vi "FS Operation Variable.vi"(9 "Variable":T1, 11 "Feature In":string="FeatureScript 1247;\nimport(path : \"onshape/std/geometry.fs\", version : \"1247.0\");\n\nannotation { \"Feature Type Name\" : \"LabVIEW Feature\" }\nexport const myFeature = defineFeature(function(context is Context, id is Id, definition is map)\n    precondition\n    {\n        // Define the parameters of the feature type\n    }\n    {\n        // Define the function's action\n    });") -> (3 "Feature Out":string="FeatureScript 1247;\nimport(path : \"onshape/std/geometry.fs\", version : \"1247.0\");\n\nannotation { \"Feature Type Name\" : \"LVFeat1\" }\nexport const myFeature = defineFeature(function(context is Context, id is Id, definition is map)\n    precondition\n    {\n        // Define the parameters of the feature type\n    }\n    {\n        // Define the function's action\n\nvar sketch1 = newSketch(context, id + \"sketch1\", {\n                \"sketchPlane\" : qCreatedBy(makeId(\"Top\"), EntityType.FACE)\n        });\n        // Create sketch entities here\n        skRectangle(sketch1, \"rectangle1\", {\n                \"firstCorner\" : vector(0, 0) * inch,\n                \"secondCorner\" : vector(3, 4) * inch\n        });\n        \n        skSolve(sketch1);\n    });")   [LabVIEW 2019]
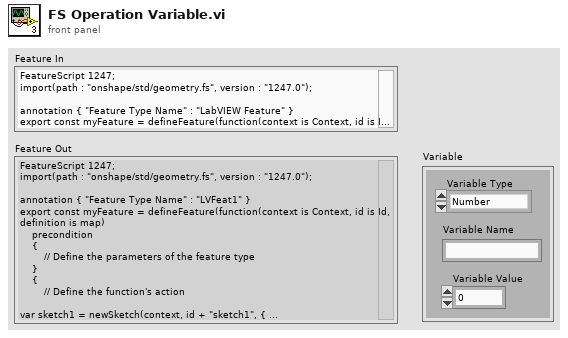
[diagram p1: front panel]
types:
  T1 = cluster{"Variable Type":enum16{"Number", "Length", "Angle", "Any"}, "Variable Name":string, "Variable Value":dbl}
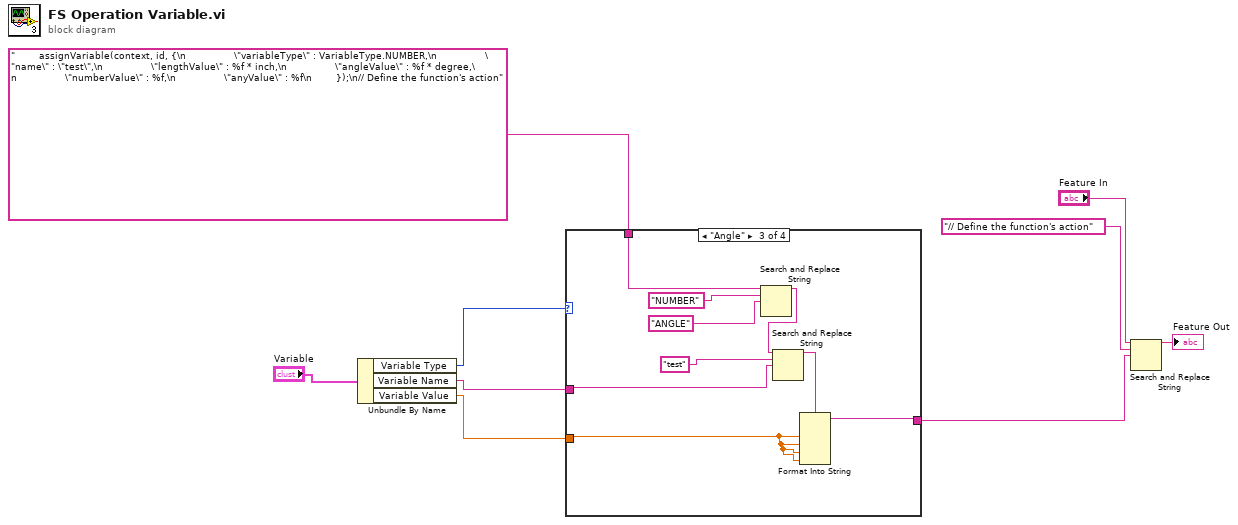
[diagram p0: block diagram]
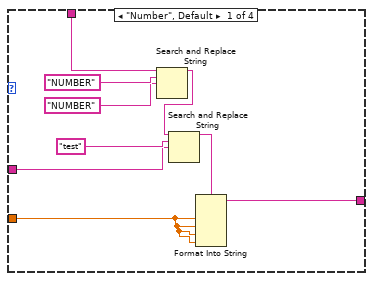
[diagram p2: hidden frame]
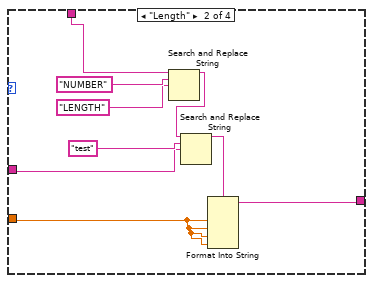
[diagram p3: hidden frame]
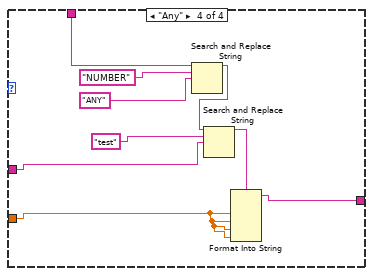
[diagram p4: hidden frame]
diagram:
  n1 = Unbundle By Name("Variable") -> ("Variable Type"=w5:enum16{"Number", "Length", "Angle", "Any"}, "Variable Name"=w3:string, "Variable Value"=w2:dbl)
  n2 = case shown="\"Angle\"" w5 {
    tunnel: "        assignVariable(context, id, {\n                \"variableType\" : VariableType.NUMBER,\n                \"name\" : \"test\",\n                \"lengthValue\" : %f * inch,\n                \"angleValue\" : %f * degree,\n                \"numberValue\" : %f,\n                \"anyValue\" : %f\n        });\n// Define the function's action" ("search string") -> [w18 w20 w31 w40]
    tunnel: w3 -> [w13 w21 w30 w39]
    tunnel: w2 -> [w12 w22 w29 w38]
    tunnel: [w10 w19 w28 w37] -> w1
    frame "Number", Default {
      n3 = Search and Replace String(input string=w18, search string="NUMBER", replace string="NUMBER") -> (result string=w14:string)  [unwired: 5 in, 3 out]
      n4 = Search and Replace String(input string=w14, search string="test", replace string=w13) -> (result string=w11:string)  [unwired: 5 in, 3 out]
      n5 = Format Into String(format string=w11, w12, w12, w12, w12) -> (resulting string=w10:string)  [unwired: 2 in, 1 out]
    }
    frame "Length" {
      n6 = Search and Replace String(input string=w20, search string="NUMBER", replace string="LENGTH") -> (result string=w24:string)  [unwired: 5 in, 3 out]
      n7 = Search and Replace String(input string=w24, search string="test", replace string=w21) -> (result string=w23:string)  [unwired: 5 in, 3 out]
      n8 = Format Into String(format string=w23, w22, w22, w22, w22) -> (resulting string=w19:string)  [unwired: 2 in, 1 out]
    }
    frame "Angle" {
      n9 = Search and Replace String(input string=w31, search string="NUMBER", replace string="ANGLE") -> (result string=w35:string)  [unwired: 5 in, 3 out]
      n10 = Search and Replace String(input string=w35, search string="test", replace string=w30) -> (result string=w36:string)  [unwired: 5 in, 3 out]
      n11 = Format Into String(format string=w36, w29, w29, w29, w29) -> (resulting string=w28:string)  [unwired: 2 in, 1 out]
    }
    frame "Any" {
      n12 = Search and Replace String(input string=w40, search string="NUMBER", replace string="ANY") -> (result string=w44:string)  [unwired: 5 in, 3 out]
      n13 = Search and Replace String(input string=w44, search string="test", replace string=w39) -> (result string=w45:string)  [unwired: 5 in, 3 out]
      n14 = Format Into String(format string=w45, w38, w38, w38, w38) -> (resulting string=w37:string)  [unwired: 2 in, 1 out]
    }
  }
  n15 = Search and Replace String(input string="Feature In", search string="// Define the function's action", replace string=w1) -> (result string=→"Feature Out":string)  [unwired: 5 in, 3 out]
